vi "cRIO_main.vi"() -> ()   [LabVIEW 2014]
uses:
  System_States.ctl
  Timer 2013/Control Timer.ctl
  <vilib>/functionblocks/Edge Detection/One Shot Rising with Input/One Shot Rising with Input.vi
  <vilib>/functionblocks/Edge Detection/One Shot Falling With Input/One Shot Falling With Input.vi
  <vilib>/functionblocks/FB Core/FB Core.xnode
  <vilib>/functionblocks/NI_FunctionBlock Libraries.lvlib
panel:
  out "Enum":T1
  out "Error Out":errorcluster
  in  "Error In":errorcluster
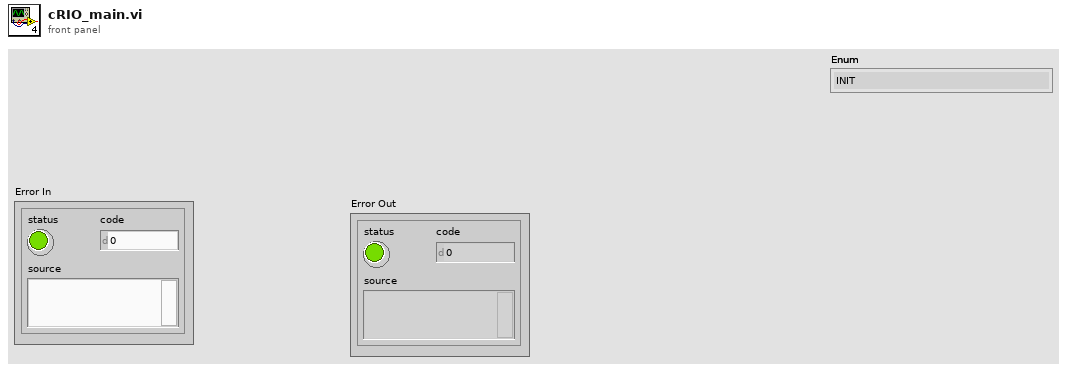
[diagram p1: front panel]
types:
  T1 = typedef "System_States.ctl" = enum16{"INIT", "IDLE", "AUTO_RUN", "AUTO_SHUTDOWN", "MANUAL_MODE", "FAULT_EMERGENCY", "FAULT"}
  T2 = typedef "Control Timer.ctl" = enum16{"Timecheck", "Reset"}
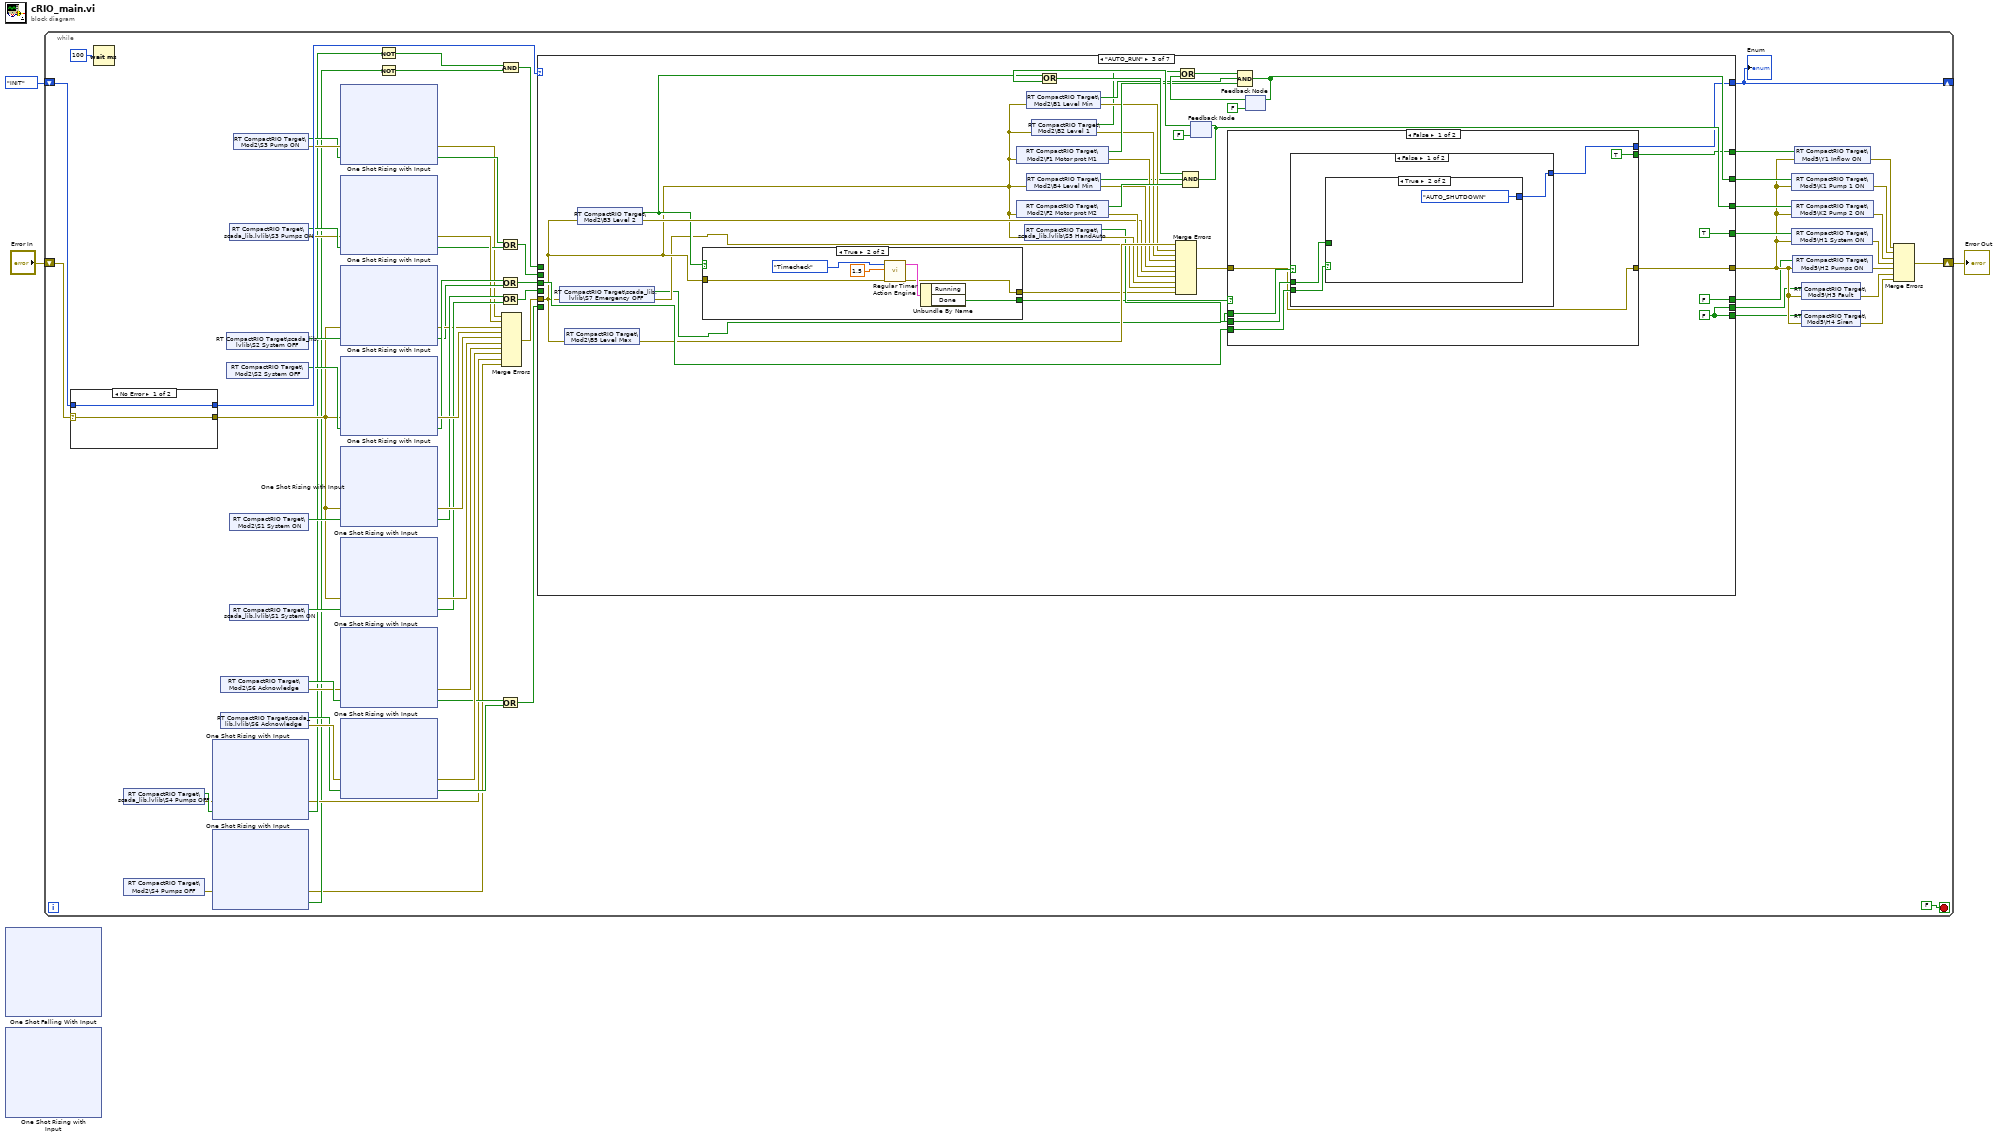
[diagram p0: block diagram]
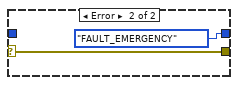
[diagram p2: hidden frame]
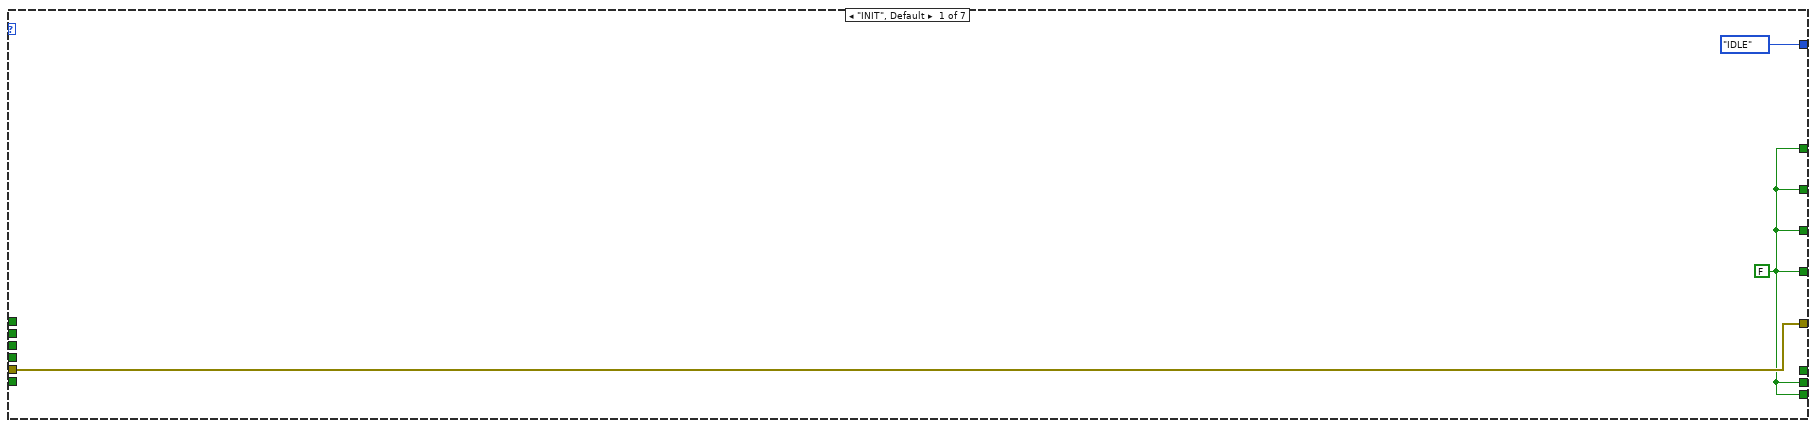
[diagram p3: hidden frame]
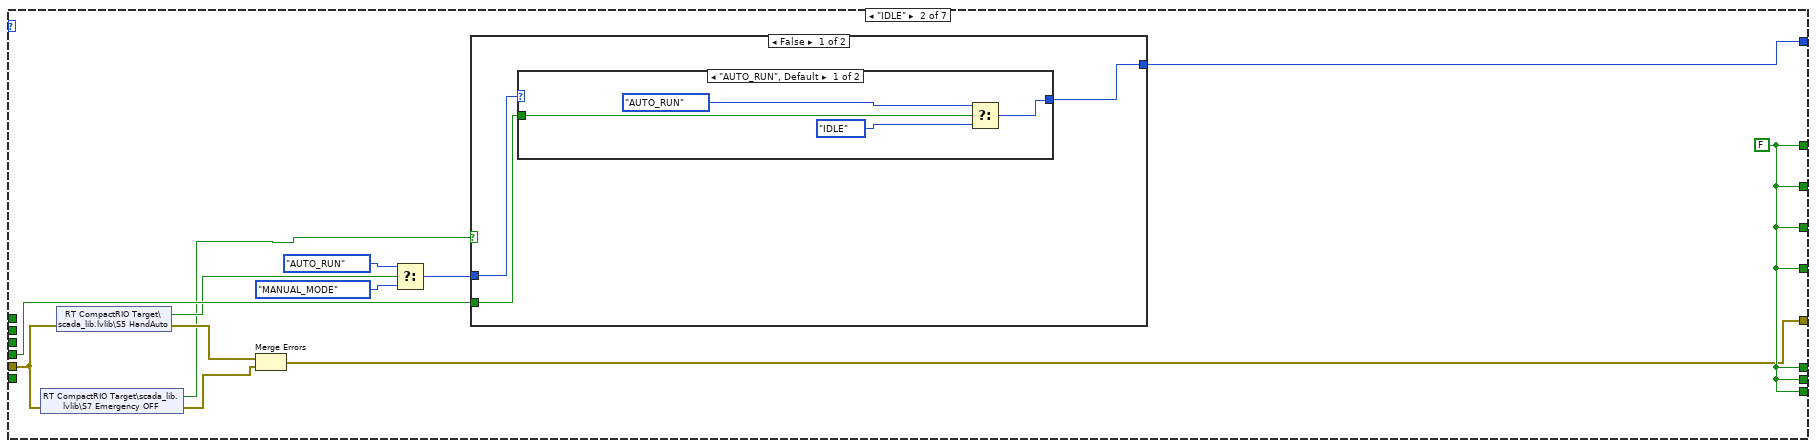
[diagram p4: hidden frame]
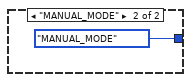
[diagram p5: hidden frame]
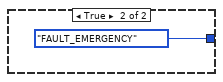
[diagram p6: hidden frame]
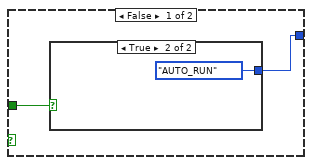
[diagram p7: hidden frame]
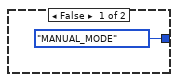
[diagram p8: hidden frame]
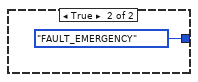
[diagram p9: hidden frame]
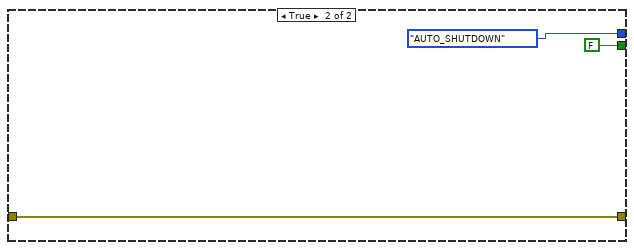
[diagram p10: hidden frame]
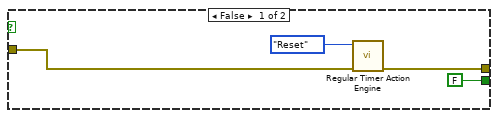
[diagram p11: hidden frame]
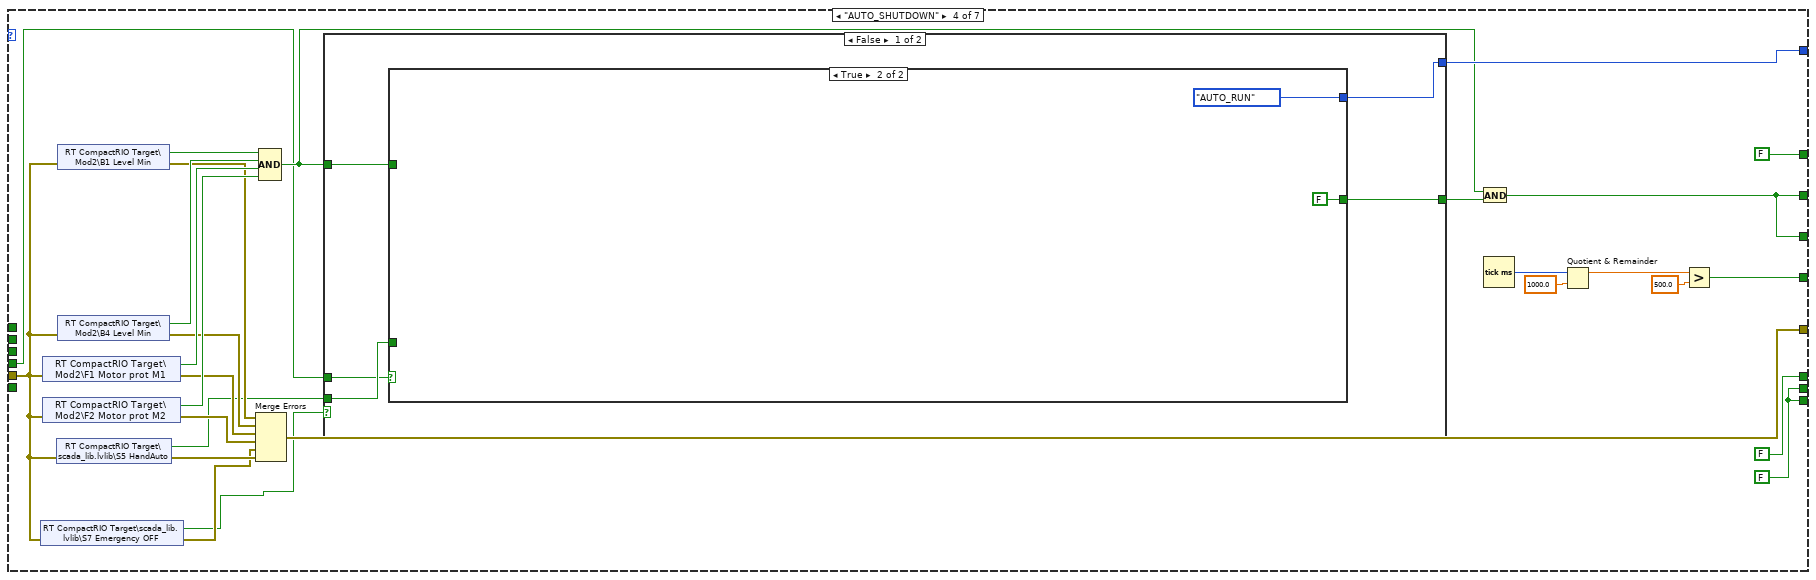
[diagram p12: hidden frame]
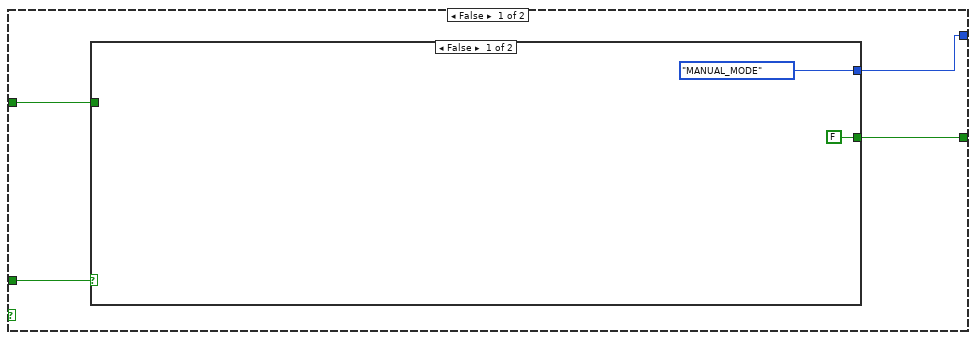
[diagram p13: hidden frame]
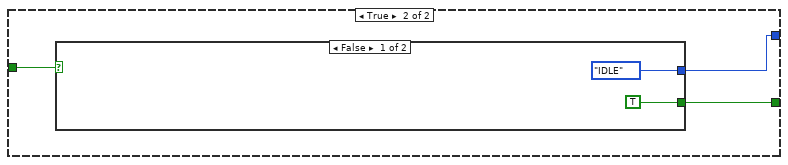
[diagram p14: hidden frame]
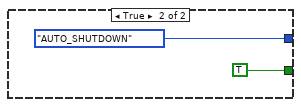
[diagram p15: hidden frame]
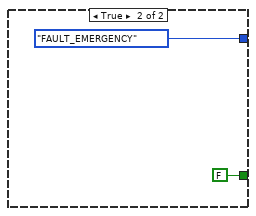
[diagram p16: hidden frame]
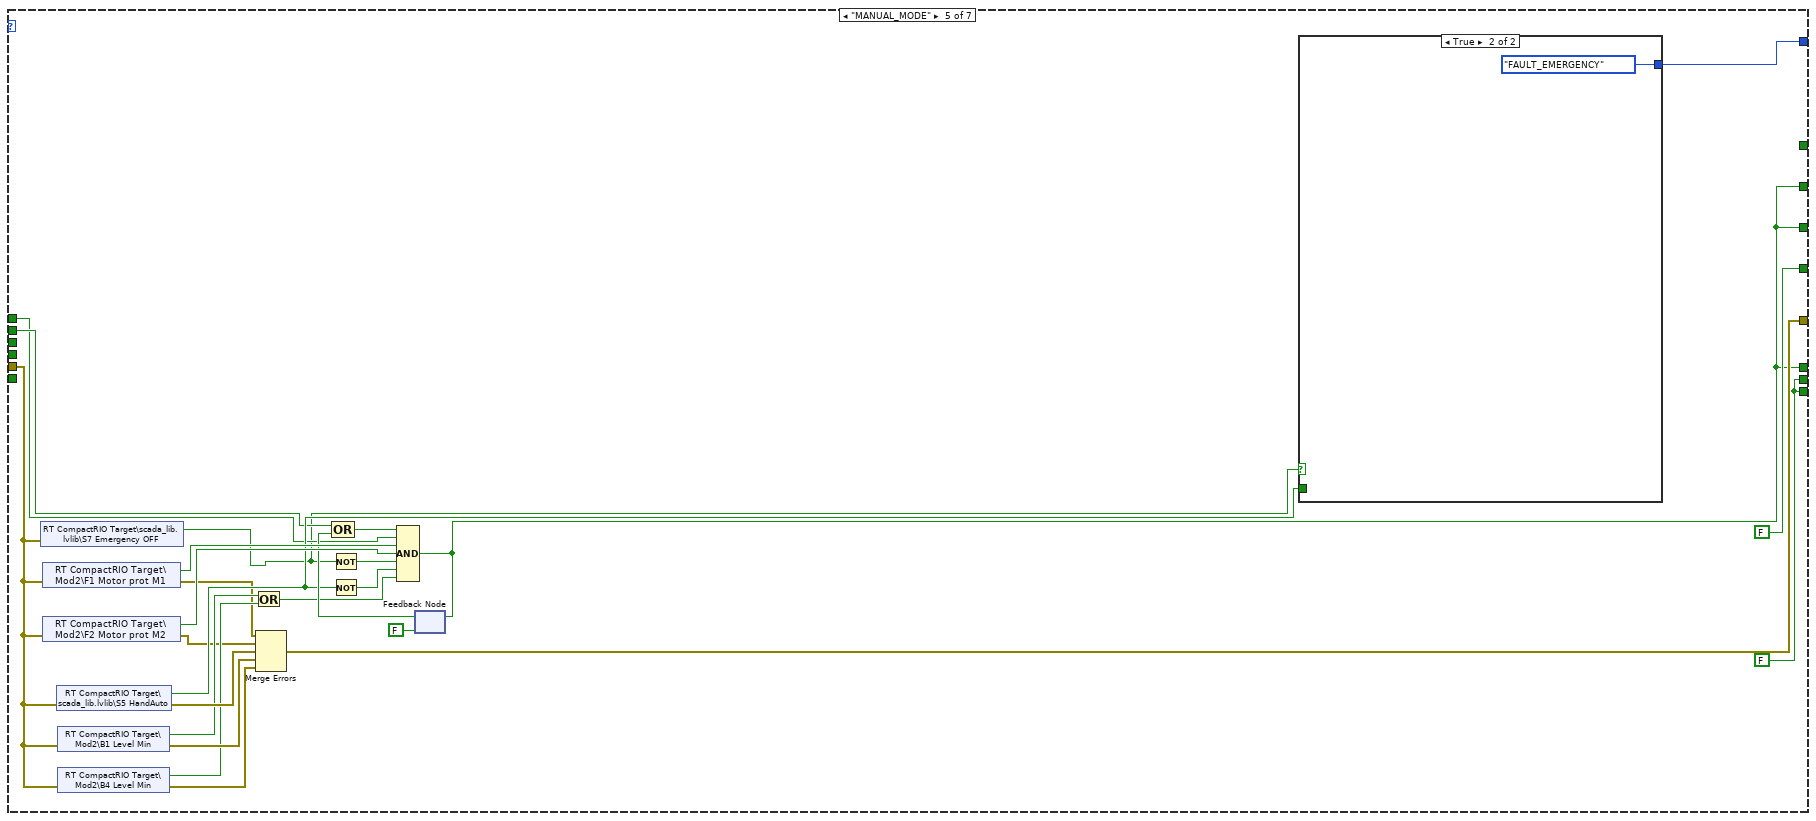
[diagram p17: hidden frame]
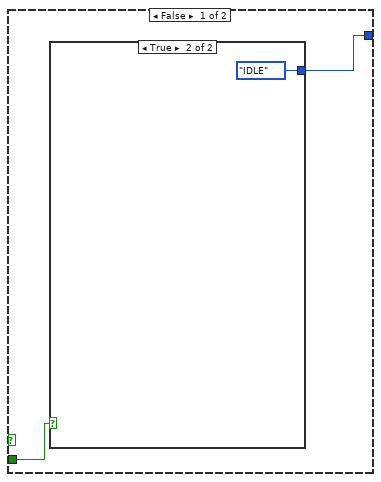
[diagram p18: hidden frame]
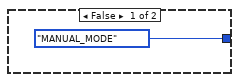
[diagram p19: hidden frame]
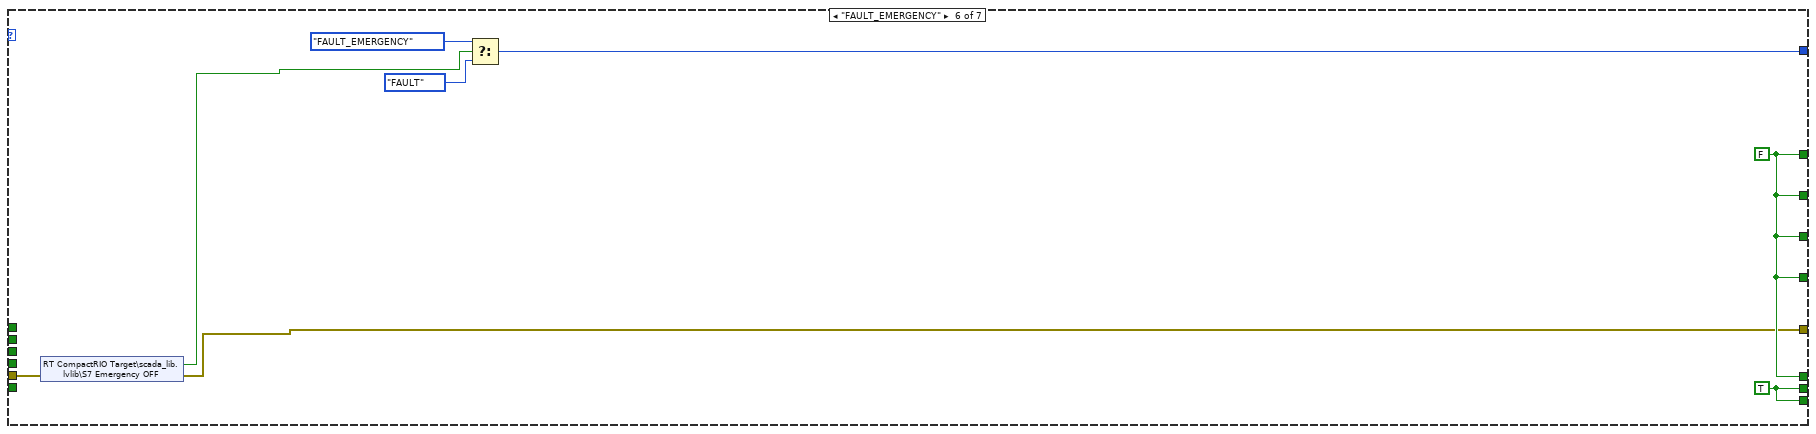
[diagram p20: hidden frame]
diagram:
  n1 = xnode "One Shot Falling With Input"() -> ()  [unwired: 2 in, 2 out]
  n2 = xnode "One Shot Rising with Input"() -> ()  [unwired: 2 in, 2 out]
  n3 = while {
    shift-right: [w52] -> _
    shift-left: System_States."INIT" -> [w64]
    shift-right: [w53] -> w1
    shift-left: "Error In" -> [w69]
    stop <- FALSE stop-if-true
    n4 = case shown="No Error" w69 {
      selector: w69 -> [w449 w450]
      tunnel: [w449 w450] -> w35
      tunnel: w64 -> [w448 _]
      tunnel: [w448 System_States."FAULT_EMERGENCY"] -> w63
      frame No Error {
      }
      frame Error {
      }
    }
    n5 = Wait (ms)(milliseconds to wait=u32 100) -> ()  [unwired: 1 out]
    n6 = shared-variable "RT CompactRIO Target\\scada_lib.lvlib\\S4 Pumps OFF"() -> (w13:bool, error out=w12:errorcluster)  [unwired: 1 in]
    n7 = shared-variable "RT CompactRIO Target\\Mod2\\S4 Pumps OFF"() -> (error out=w9:errorcluster)  [unwired: 1 in, 1 out]
    n8 = xnode "One Shot Rising with Input"("error in"=w12, "input"=w13) -> ("error out"=w10:errorcluster, "output"=w11:bool)
    n9 = xnode "One Shot Rising with Input"("error in"=w9) -> ("error out"=w7:errorcluster, "output"=w8:bool)  [unwired: 1 in]
    n10 = shared-variable "RT CompactRIO Target\\Mod2\\S6 Acknowledge"() -> (w29:bool, error out=w28:errorcluster)  [unwired: 1 in]
    n11 = shared-variable "RT CompactRIO Target\\scada_lib.lvlib\\S6 Acknowledge"() -> (w30:bool, error out=w31:errorcluster)  [unwired: 1 in]
    n12 = shared-variable "RT CompactRIO Target\\scada_lib.lvlib\\S2 System OFF"() -> (w36:bool)  [unwired: 1 in, 1 out]
    n13 = shared-variable "RT CompactRIO Target\\Mod2\\S2 System OFF"() -> (w44:bool)  [unwired: 1 in, 1 out]
    n14 = shared-variable "RT CompactRIO Target\\scada_lib.lvlib\\S3 Pumps ON"() -> (w22:bool, error out=w21:errorcluster)  [unwired: 1 in]
    n15 = shared-variable "RT CompactRIO Target\\Mod2\\S1 System ON"() -> (w51:bool)  [unwired: 1 in, 1 out]
    n16 = shared-variable "RT CompactRIO Target\\scada_lib.lvlib\\S1 System ON"() -> (w41:bool)  [unwired: 1 in, 1 out]
    n17 = shared-variable "RT CompactRIO Target\\Mod2\\S3 Pump ON"() -> (w18:bool, error out=w19:errorcluster)  [unwired: 1 in]
    n18 = xnode "One Shot Rising with Input"("error in"=w19, "input"=w18) -> ("error out"=w14:errorcluster, "output"=w15:bool)
    n19 = xnode "One Shot Rising with Input"("error in"=w21, "input"=w22) -> ("error out"=w20:errorcluster, "output"=w17:bool)
    n20 = xnode "One Shot Rising with Input"("error in"=w35, "input"=w36) -> ("error out"=w34:errorcluster, "output"=w32:bool)
    n21 = xnode "One Shot Rising with Input"("error in"=w35, "input"=w44) -> ("error out"=w43:errorcluster, "output"=w42:bool)
    n22 = xnode "One Shot Rising with Input"("error in"=w35, "input"=w51) -> ("error out"=w49:errorcluster, "output"=w39:bool)
    n23 = xnode "One Shot Rising with Input"("error in"=w35, "input"=w41) -> ("error out"=w40:errorcluster, "output"=w37:bool)
    n24 = xnode "One Shot Rising with Input"("error in"=w28, "input"=w29) -> ("error out"=w27:errorcluster, "output"=w25:bool)
    n25 = xnode "One Shot Rising with Input"("error in"=w31, "input"=w30) -> ("error out"=w26:errorcluster, "output"=w24:bool)
    n26 = Not(x=w11) -> (.not. x?=w6:bool)
    n27 = Not(x=w8) -> (.not. x?=w5:bool)
    n28 = Or(x=w15, y=w17) -> (x .or. y?=w16:bool)
    n29 = Or(x=w42, y=w32) -> (x .or. y?=w33:bool)
    n30 = Or(x=w39, y=w37) -> (x .or. y?=w38:bool)
    n31 = Or(x=w25, y=w24) -> (x .or. y?=w23:bool)
    n32 = And(x=w6, y=w5) -> (x .and. y?=w4:bool)
    n33 = Merge Errors(w14, w20, w34, w43, w49, w40, w27, w26, w10, w7) -> (w48:errorcluster)
    n34 = case shown="\"AUTO_RUN\"" w63 {
      tunnel: [System_States."IDLE" w465 w500 w556 w606 w624 w629] -> w52
      tunnel: [w452 w461 w480 FALSE _ w623 w632] -> w68
      tunnel: [w452 w461 w509 w546 w604 w623 w632] -> w67
      tunnel: [w452 w461 w503 w546 w604 w623 w632] -> w66
      tunnel: [w452 w461 TRUE w561 FALSE w623 w632] -> w65
      tunnel: [w452 w461 w495 w555 w607 w622 w633] -> w45
      tunnel: w48 -> [w453 w459 w482 w543 w602 w621 w628]
      tunnel: [w453 w460 w478 w549 w605 w619 w628] -> w61
      tunnel: w38 -> [_ w462 _ w542 _ _ _]
      tunnel: w33 -> [_ _ w499 _ _ _ _]
      tunnel: [w452 w461 w495 w555 w607 w622 w633] -> w47
      tunnel: [_ w461 FALSE FALSE w604 w623 w632] -> w46
      tunnel: w23 -> [_ _ _ _ _ _ w627]
      tunnel: w16 -> [_ _ _ _ w594 _ _]
      tunnel: w4 -> [_ _ _ _ w593 _ _]
      frame "INIT", Default {
        w452 = FALSE
      }
      frame "IDLE" {
        w461 = FALSE
        n35 = shared-variable "RT CompactRIO Target\\scada_lib.lvlib\\S7 Emergency OFF"(error in=w459) -> (w456:bool, error out=w455:errorcluster)
        n36 = shared-variable "RT CompactRIO Target\\scada_lib.lvlib\\S5 HandAuto"(error in=w459) -> (w458:bool, error out=w457:errorcluster)
        n37 = Merge Errors(w457, w455) -> (w460:errorcluster)
        n38 = Select(t=System_States."AUTO_RUN", s=w458, f=System_States."MANUAL_MODE") -> (s? t:f=w466:T1)
        n39 = case shown="False" w456 {
          tunnel: w466 -> [w469 _]
          tunnel: [w468 System_States."FAULT_EMERGENCY"] -> w465
          tunnel: w462 -> [w467 _]
          frame False {
            n40 = case shown="\"AUTO_RUN\", Default" w469 {
              tunnel: [w472 System_States."MANUAL_MODE"] -> w468
              tunnel: w467 -> [w471 _]
              frame "AUTO_RUN", Default {
                n41 = Select(t=System_States."AUTO_RUN", s=w471, f=System_States."IDLE") -> (s? t:f=w472:T1)
              }
              frame "MANUAL_MODE" {
              }
            }
          }
          frame True {
          }
        }
      }
      frame "AUTO_RUN" {
        w495 = FALSE
        n42 = shared-variable "RT CompactRIO Target\\scada_lib.lvlib\\S7 Emergency OFF"(error in=w482) -> (w476:bool, error out=w477:errorcluster)
        n43 = shared-variable "RT CompactRIO Target\\Mod2\\B5 Level Max"(error in=w482) -> (error out=w498:errorcluster)  [unwired: 1 out]
        n44 = shared-variable "RT CompactRIO Target\\Mod2\\B3 Level 2"(error in=w482) -> (w484:bool, error out=w485:errorcluster)
        n45 = case shown="True" w484 {
          tunnel: [FALSE w536] -> w483
          tunnel: w482 -> [w531 w535]
          tunnel: [w530 w534] -> w481
          frame False {
            n46 = call "Regular Timer Action Engine.vi"("Enum"=Control_Timer."Reset", "error in"=w531) -> ("error out"=w530:errorcluster)  [unwired: 7 in, 1 out]
          }
          frame True {
            n47 = call "Regular Timer Action Engine.vi"("Enum"=Control_Timer."Timecheck", "Time Target"=1.5, "error in"=w535) -> ("Status"=w537:cluster{"Running":bool, "Done":bool}, "error out"=w534:errorcluster)  [unwired: 6 in]
            n48 = Unbundle By Name(w537) -> ("Done"=w536:bool)  [unwired: 1 out]
          }
        }
        n49 = shared-variable "RT CompactRIO Target\\Mod2\\F1 Motor prot M1"(error in=w482) -> (w502:bool, error out=w497:errorcluster)
        n50 = shared-variable "RT CompactRIO Target\\Mod2\\F2 Motor prot M2"(error in=w482) -> (w501:bool, error out=w496:errorcluster)
        n51 = shared-variable "RT CompactRIO Target\\scada_lib.lvlib\\S5 HandAuto"(error in=w482) -> (w492:bool, error out=w493:errorcluster)
        n52 = shared-variable "RT CompactRIO Target\\Mod2\\B1 Level Min"(error in=w482) -> (w490:bool, error out=w491:errorcluster)
        n53 = shared-variable "RT CompactRIO Target\\Mod2\\B4 Level Min"(error in=w482) -> (w486:bool, error out=w487:errorcluster)
        n54 = shared-variable "RT CompactRIO Target\\Mod2\\B2 Level 1"(error in=w482) -> (w488:bool, error out=w489:errorcluster)
        n55 = Merge Errors(w498, w491, w489, w497, w487, w485, w496, w493, w477, w481) -> (w479:errorcluster)
        n56 = feedback #1(FALSE) -> (w505:bool)
        n57 = Or(x=w484, y=w505) -> (x .or. y?=w506:bool)
        n58 = Compound Arithmetic op=AND(w506, w486, w501) -> (w503:bool)
        n59 = feedback-in #1(w503) -> ()
        n60 = case shown="False" w483 {
          tunnel: [w517 System_States."AUTO_SHUTDOWN"] -> w500
          tunnel: w499 -> [w516 _]
          tunnel: w476 -> [w515 _]
          tunnel: w492 -> [w514 _]
          tunnel: [TRUE FALSE] -> w480
          tunnel: w479 -> [w512 w527]
          tunnel: [w512 w527] -> w478
          frame False {
            n61 = case shown="False" w515 {
              tunnel: [w519 System_States."FAULT_EMERGENCY"] -> w517
              tunnel: w516 -> [w520 _]
              tunnel: w514 -> [w518 _]
              frame False {
                n62 = case shown="True" w520 {
                  tunnel: [w521 System_States."AUTO_SHUTDOWN"] -> w519
                  tunnel: w518 -> [w522 _]
                  frame False {
                    n63 = case shown="True" w522 {
                      tunnel: [System_States."MANUAL_MODE" System_States."AUTO_RUN"] -> w521
                      frame False {
                      }
                      frame True {
                      }
                    }
                  }
                  frame True {
                  }
                }
              }
              frame True {
              }
            }
          }
          frame True {
          }
        }
        n64 = feedback #2(FALSE) -> (w508:bool)
        n65 = Or(x=w488, y=w508) -> (x .or. y?=w510:bool)
        n66 = Compound Arithmetic op=AND(w510, w490, w502) -> (w509:bool)
        n67 = feedback-in #2(w509) -> ()
      }
      frame "AUTO_SHUTDOWN" {
        w555 = FALSE
        n68 = shared-variable "RT CompactRIO Target\\scada_lib.lvlib\\S7 Emergency OFF"(error in=w543) -> (w540:bool, error out=w541:errorcluster)
        n69 = shared-variable "RT CompactRIO Target\\Mod2\\F1 Motor prot M1"(error in=w543) -> (w558:bool, error out=w551:errorcluster)
        n70 = shared-variable "RT CompactRIO Target\\Mod2\\F2 Motor prot M2"(error in=w543) -> (w557:bool, error out=w550:errorcluster)
        n71 = shared-variable "RT CompactRIO Target\\scada_lib.lvlib\\S5 HandAuto"(error in=w543) -> (w547:bool, error out=w548:errorcluster)
        n72 = shared-variable "RT CompactRIO Target\\Mod2\\B1 Level Min"(error in=w543) -> (w560:bool, error out=w553:errorcluster)
        n73 = shared-variable "RT CompactRIO Target\\Mod2\\B4 Level Min"(error in=w543) -> (w559:bool, error out=w552:errorcluster)
        n74 = Merge Errors(w553, w552, w551, w550, w541, w548) -> (w549:errorcluster)
        n75 = Compound Arithmetic op=AND(w560, w559, w558, w557) -> (w545:bool)
        n76 = case shown="False" w540 {
          tunnel: [w570 System_States."FAULT_EMERGENCY"] -> w556
          tunnel: w545 -> [w571 _]
          tunnel: w547 -> [w569 _]
          tunnel: [w568 FALSE] -> w544
          tunnel: w542 -> [w567 _]
          frame False {
            n77 = case shown="True" w567 {
              tunnel: w571 -> [w575 _]
              tunnel: [w574 System_States."AUTO_RUN"] -> w570
              tunnel: w569 -> [w573 _]
              tunnel: [w572 FALSE] -> w568
              frame False {
                n78 = case shown="False" w573 {
                  tunnel: w575 -> [_ w580]
                  tunnel: [System_States."MANUAL_MODE" w579] -> w574
                  tunnel: [FALSE w578] -> w572
                  frame False {
                  }
                  frame True {
                    n79 = case shown="False" w580 {
                      tunnel: [System_States."IDLE" System_States."AUTO_SHUTDOWN"] -> w579
                      tunnel: [TRUE TRUE] -> w578
                      frame False {
                      }
                      frame True {
                      }
                    }
                  }
                }
              }
              frame True {
              }
            }
          }
          frame True {
          }
        }
        n80 = And(x=w545, y=w544) -> (x .and. y?=w546:bool)
        n81 = Tick Count (ms)() -> (millisecond timer value=w566:u32)
        n82 = Quotient & Remainder(x=w566, y=1000.0) -> (x-y*floor(x/y)=w564:dbl)  [unwired: 1 out]
        n83 = Greater?(x=w564, y=500.0) -> (0:w561:bool)
      }
      frame "MANUAL_MODE" {
        w607 = FALSE
        n84 = shared-variable "RT CompactRIO Target\\scada_lib.lvlib\\S7 Emergency OFF"(error in=w602) -> (w591:bool)  [unwired: 1 out]
        n85 = shared-variable "RT CompactRIO Target\\Mod2\\F1 Motor prot M1"(error in=w602) -> (w612:bool, error out=w589:errorcluster)
        n86 = shared-variable "RT CompactRIO Target\\Mod2\\F2 Motor prot M2"(error in=w602) -> (w611:bool, error out=w590:errorcluster)
        n87 = shared-variable "RT CompactRIO Target\\scada_lib.lvlib\\S5 HandAuto"(error in=w602) -> (w600:bool, error out=w603:errorcluster)
        n88 = shared-variable "RT CompactRIO Target\\Mod2\\B1 Level Min"(error in=w602) -> (w597:bool, error out=w598:errorcluster)
        n89 = shared-variable "RT CompactRIO Target\\Mod2\\B4 Level Min"(error in=w602) -> (w595:bool, error out=w596:errorcluster)
        n90 = Or(x=w597, y=w595) -> (x .or. y?=w592:bool)
        n91 = Merge Errors(w589, w590, w603, w598, w596) -> (w605:errorcluster)
        n92 = Not(x=w591) -> (.not. x?=w601:bool)
        n93 = Not(x=w600) -> (.not. x?=w599:bool)
        n94 = feedback #3(FALSE) -> (w610:bool)
        n95 = Compound Arithmetic op=OR(w594, w610) -> (w613:bool)
        n96 = Compound Arithmetic op=AND(w613, w593, w612, w611, w601, w599, w592) -> (w604:bool)
        n97 = feedback-in #3(w604) -> ()
        n98 = case shown="True" w591 {
          tunnel: [w614 System_States."FAULT_EMERGENCY"] -> w606
          tunnel: w600 -> [w615 _]
          frame False {
            n99 = case shown="True" w615 {
              tunnel: [System_States."MANUAL_MODE" System_States."IDLE"] -> w614
              frame False {
              }
              frame True {
              }
            }
          }
          frame True {
          }
        }
      }
      frame "FAULT_EMERGENCY" {
        w622 = TRUE
        w623 = FALSE
        n100 = shared-variable "RT CompactRIO Target\\scada_lib.lvlib\\S7 Emergency OFF"(error in=w621) -> (w620:bool, error out=w619:errorcluster)
        n101 = Select(t=System_States."FAULT_EMERGENCY", s=w620, f=System_States."FAULT") -> (s? t:f=w624:T1)
      }
      frame "FAULT" {
        w632 = FALSE
        w633 = TRUE
        n102 = Select(t=System_States."IDLE", s=w627, f=System_States."FAULT") -> (s? t:f=w629:T1)
      }
    }
    "Enum" <- w52
    n103 = shared-variable "RT CompactRIO Target\\Mod5\\K1 Pump 1 ON"(w67, error in=w61) -> (error out=w59:errorcluster)
    n104 = shared-variable "RT CompactRIO Target\\Mod5\\K2 Pump 2 ON"(w66, error in=w61) -> (error out=w58:errorcluster)
    n105 = shared-variable "RT CompactRIO Target\\Mod5\\H1 System ON"(w65, error in=w61) -> (error out=w57:errorcluster)
    n106 = shared-variable "RT CompactRIO Target\\Mod5\\H2 Pumps ON"(w46, error in=w61) -> (error out=w56:errorcluster)
    n107 = shared-variable "RT CompactRIO Target\\Mod5\\Y1 Inflow ON"(w68, error in=w61) -> (error out=w60:errorcluster)
    n108 = shared-variable "RT CompactRIO Target\\Mod5\\H3 Fault"(w45, error in=w61) -> (error out=w55:errorcluster)
    n109 = shared-variable "RT CompactRIO Target\\Mod5\\H4 Siren"(w47, error in=w61) -> (error out=w54:errorcluster)
    n110 = Merge Errors(w60, w59, w58, w57, w56, w55, w54) -> (w53:errorcluster)
  }
  "Error Out" <- w1
